vi "LevMar - TestSuite - Function.vi"(1 "A":dbl[](array[numeric])) -> (0 "F":dbl[](array[numeric]))   [LabVIEW 2009]
panel:
  in  "X":dbl[](array[numeric])
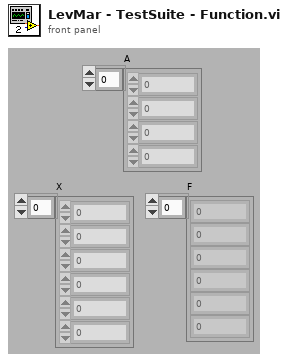
[diagram p1: front panel]
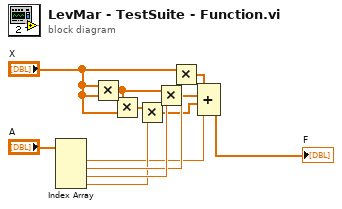
[diagram p0: block diagram]
diagram:
  n1 = Index Array(array="A") -> (element #1=w1:dbl, element #2=w10:dbl, element #3=w11:dbl, element #4=w3:dbl)  [unwired: 4 in]
  n2 = Multiply(x="X", y="X") -> (x*y=w6:dbl[])
  n3 = Multiply(x=w6, y="X") -> (x*y=w4:dbl[])
  n4 = Multiply(x=w4, y=w3) -> (x*y=w2:dbl[])
  n5 = Multiply(x=w6, y=w11) -> (x*y=w9:dbl[])
  n6 = Multiply(x="X", y=w10) -> (x*y=w8:dbl[])
  n7 = Compound Arithmetic op=ADD(w8, w9, w2, w1) -> (→"F":dbl[])
